vi "Configure MFC.vi"(7 "MFC Mode (0: Voltage)":u16(ring) items=["Voltage", "Current"], 8 "error in (no error)":errorcluster, 9 "MFC Channel (1: Channel 1)":i32(ring)=1 items=["Channel 1"=1, "Channel 2"=2, "Channel 3"=3, "Channel 4"=4, "Channel 5"=5], 10 "Enable MFC (Enable)":bool=TRUE, 11 "VISA resource name":refnum<visa-resource-name>) -> (0 "error out":errorcluster, 3 "VISA resource name out":refnum<visa-resource-name>)   [LabVIEW 2023, in "Fluke Molbox 1 Plus.lvlib"]
doc: "Configures the MFC channel and output mode. The optional MFC interface can support voltage or current controlled MFC's. There is also an available MFC switchbox, which is controlled by the molbox1+."
uses:
  Fluke Molbox 1 Plus.lvlib
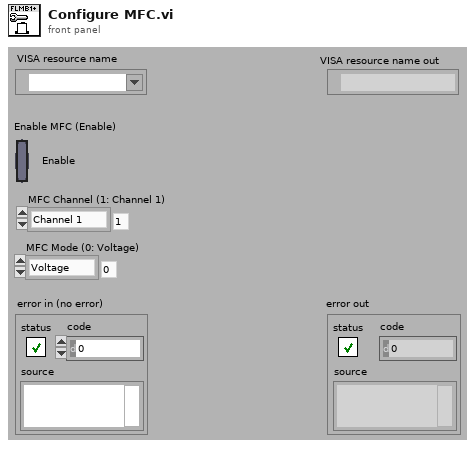
[diagram p1: front panel]
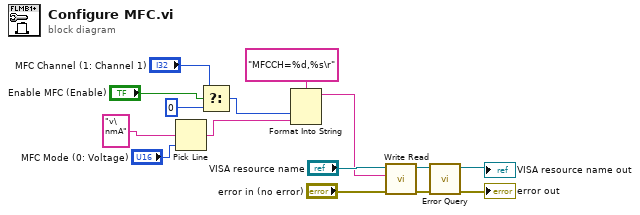
[diagram p0: block diagram]
diagram:
  n1 = Pick Line(multi-line string="v\nmA", line index="MFC Mode (0: Voltage)") -> (output string=w12:string)  [unwired: 1 in]
  n2 = Select(t="MFC Channel (1: Channel 1)", s="Enable MFC (Enable)", f=0) -> (s? t:f=w11:i32)
  n3 = Format Into String(format string="MFCCH=%d,%s\r", w11, w12) -> (resulting string=w6:string)  [unwired: 2 in, 1 out]
  n4 = call "Write Read.vi"("error in (no error)"="error in (no error)", "Write String"=w6, "VISA resource name"="VISA resource name") -> ("error out"=w3:errorcluster, "VISA resource name out"=w4:refnum<visa-resource-name>)  [unwired: 6 in, 1 out]
  n5 = call "Error Query.vi"("error in (no error)"=w3, "VISA resource name"=w4) -> ("error out"=→"error out":errorcluster, "VISA resource name out"=→"VISA resource name out":refnum<visa-resource-name>)  [unwired: 6 in, 2 out]
